vi "Lift state machine.vi"(10 "Grabber Height":dbl, 11 "Joystick Buttons":T2) -> (3 "Motor speed":dbl)   [LabVIEW 2014]
uses:
  Lift state.ctl
  Joystick Buttons typedef.ctl
panel:
  in  "Level setpoints":dbl[](array[numeric])
  in  "Destination":T1
  in  "Direction":enum16{"Not in motion", "Down", "Up"}(ring)
  in  "Lift state":T1
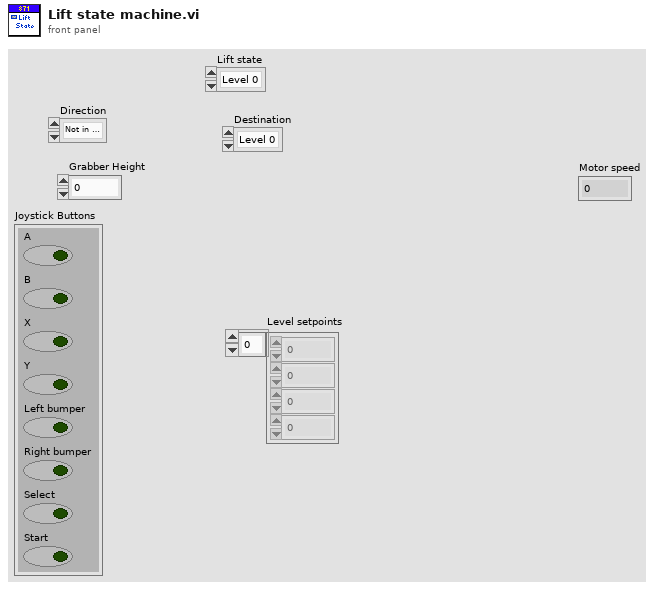
[diagram p1: front panel]
types:
  T1 = typedef "Lift state.ctl" = enum16{"Level 0", "Level 1", "Level 2", "level 3", "Placement State"}
  T2 = typedef "Joystick Buttons typedef.ctl" = cluster{"A":bool, "B":bool, "X":bool, "Y":bool, "Left bumper":bool, "Right bumper":bool, "Select":bool, "Start":bool}
  T3 = typedef "WPI_DigitalInputDevRef.ctl" = cluster{"DevStatus":errorcluster, "DIO Channel":T4, "Controller":T5}
  T4 = typedef "FPGA_DIOChannel.ctl" = enum8{"DIO 0", "DIO 1", "DIO 2", "DIO 3", "DIO 4", "DIO 5", "DIO 6", "DIO 7", "DIO 8", "DIO 9", "DIO MXP 0", "DIO MXP 1", "DIO MXP 2", "DIO MXP 3", "DIO MXP 4", "DIO MXP 5", "DIO MXP 6", "DIO MXP 7", "DIO MXP 8", "DIO MXP 9", "DIO MXP 10", "DIO MXP 11", "DIO MXP 12", "DIO MXP 13", "DIO MXP 14", "DIO MXP 15", "Invalid"}
  T5 = typedef "FPGA_TypedefDigitalModule.ctl" = enum16{"Controller 1"}
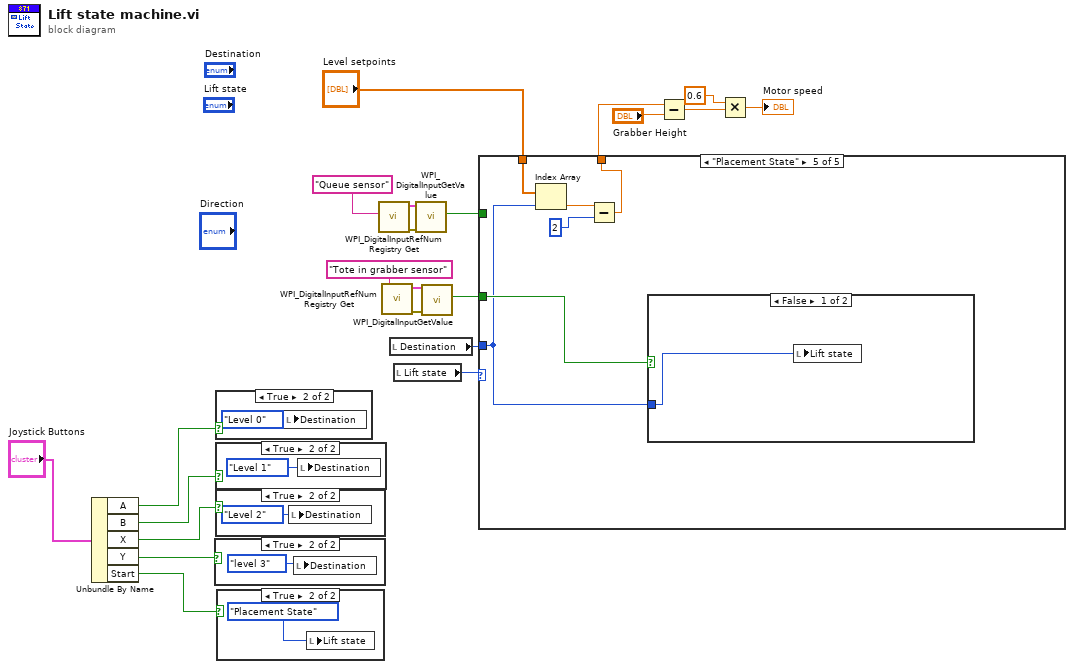
[diagram p0: block diagram]
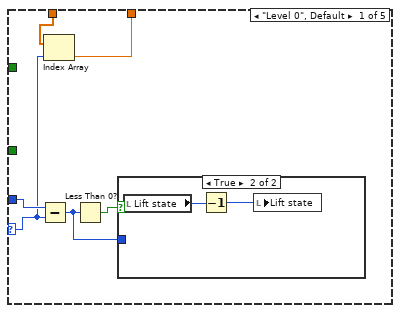
[diagram p7: hidden frame]
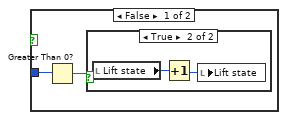
[diagram p8: hidden frame]
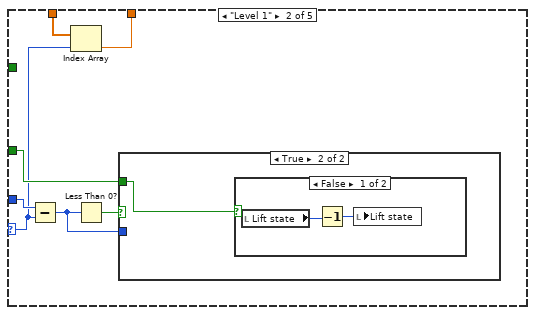
[diagram p10: hidden frame]
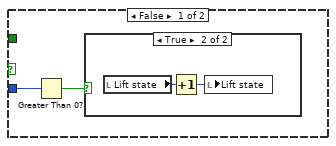
[diagram p11: hidden frame]
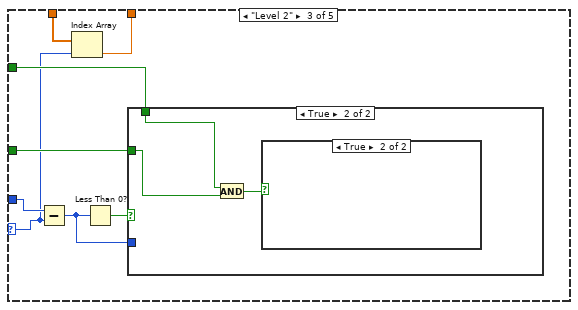
[diagram p14: hidden frame]
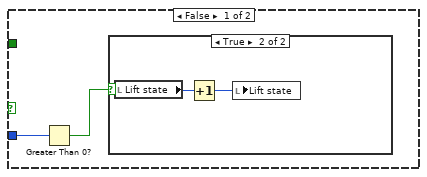
[diagram p15: hidden frame]
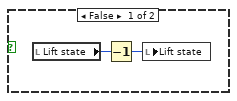
[diagram p17: hidden frame]
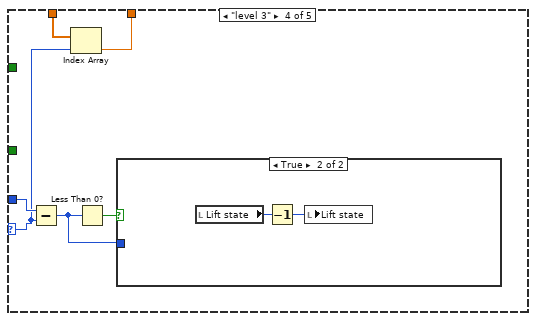
[diagram p18: hidden frame]
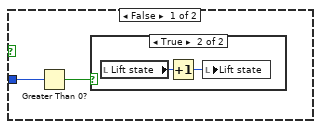
[diagram p19: hidden frame]
diagram:
  n1 = Unbundle By Name("Joystick Buttons") -> ("A"=w10:bool, "B"=w9:bool, "X"=w3:bool, "Y"=w8:bool, "Start"=w2:bool)
  n2 = case shown="True" w8 {
    frame False {
    }
    frame True {
      n3 = local write "Destination"(Lift_state."level 3" ("Lift state")) -> ()
    }
  }
  n4 = case shown="True" w10 {
    frame False {
    }
    frame True {
      n5 = local write "Destination"(Lift_state."Level 0" ("Lift state")) -> ()
    }
  }
  n6 = case shown="True" w9 {
    frame False {
    }
    frame True {
      n7 = local write "Destination"(Lift_state."Level 1" ("Lift state")) -> ()
    }
  }
  n8 = case shown="True" w3 {
    frame False {
    }
    frame True {
      n9 = local write "Destination"(Lift_state."Level 2" ("Lift state")) -> ()
    }
  }
  n10 = case shown="True" w2 {
    frame False {
    }
    frame True {
      n11 = local write "Lift state"(Lift_state."Placement State" ("Lift state")) -> ()
    }
  }
  n12 = call <vilib>:"WPI_DigitalInputRefNum Registry Get.vi"("refnum name"="Queue sensor") -> ("error out"=w7:errorcluster, "DigitalInputDevRef"=w6:T3)  [unwired: 9 in]
  n13 = call <vilib>:"WPI_DigitalInputRefNum Registry Get.vi"("refnum name"="Tote in grabber sensor") -> ("error out"=w15:errorcluster, "DigitalInputDevRef"=w14:T3)  [unwired: 9 in]
  n14 = local read "Destination"() -> (w11:T1)
  n15 = local read "Lift state"() -> (w21:T1)
  n16 = call <vilib>:"WPI_DigitalInputGetValue.vi"("error in (no error)"=w7, "DigitalInputDevRef"=w6) -> ("Value"=w4:bool)  [unwired: 7 in, 2 out]
  n17 = call <vilib>:"WPI_DigitalInputGetValue.vi"("error in (no error)"=w15, "DigitalInputDevRef"=w14) -> ("Value"=w12:bool)  [unwired: 7 in, 2 out]
  n18 = case shown="\"Placement State\"" w21 {
    selector: w21 -> [w28 w40 w54 w71 _]
    tunnel: [w30 w42 w56 w73 w85] -> w19
    tunnel: w12 -> [_ w43 w57 _ w84]
    tunnel: w11 -> [w33 w46 w59 w74 w83]
    tunnel: w4 -> [_ _ w58 _ _]
    tunnel: "Level setpoints" -> [w29 w41 w55 w72 w87]
    frame "Level 0", Default {
      n19 = Subtract(x=w33, y=w28) -> (x-y=w31:u16)
      n20 = Index Array(array=w29, index=w28) -> (element=w30:dbl)
      n21 = Less Than 0?(x=w31) -> (x < 0?=w32:bool)
      n22 = case shown="True" w32 {
        tunnel: w31 -> [w35 _]
        frame False {
          n23 = Greater Than 0?(x=w35) -> (x > 0?=w34:bool)
          n24 = case shown="True" w34 {
            frame False {
            }
            frame True {
              n25 = local read "Lift state"() -> (w37:T1)
              n26 = Increment(x=w37) -> (x+1=w36:T1)
              n27 = local write "Lift state"(w36) -> ()
            }
          }
        }
        frame True {
          n28 = local read "Lift state"() -> (w39:T1)
          n29 = Decrement(x=w39) -> (x-1=w38:T1)
          n30 = local write "Lift state"(w38) -> ()
        }
      }
    }
    frame "Level 1" {
      n31 = Subtract(x=w46, y=w40) -> (x-y=w44:u16)
      n32 = Index Array(array=w41, index=w40) -> (element=w42:dbl)
      n33 = Less Than 0?(x=w44) -> (x < 0?=w45:bool)
      n34 = case shown="True" w45 {
        tunnel: w44 -> [w48 _]
        tunnel: w43 -> [_ w51]
        frame False {
          n35 = Greater Than 0?(x=w48) -> (x > 0?=w47:bool)
          n36 = case shown="True" w47 {
            frame False {
            }
            frame True {
              n37 = local read "Lift state"() -> (w50:T1)
              n38 = Increment(x=w50) -> (x+1=w49:T1)
              n39 = local write "Lift state"(w49) -> ()
            }
          }
        }
        frame True {
          n40 = case shown="False" w51 {
            frame False {
              n41 = local read "Lift state"() -> (w53:T1)
              n42 = Decrement(x=w53) -> (x-1=w52:T1)
              n43 = local write "Lift state"(w52) -> ()
            }
            frame True {
            }
          }
        }
      }
    }
    frame "Level 2" {
      n44 = Subtract(x=w59, y=w54) -> (x-y=w60:u16)
      n45 = Index Array(array=w55, index=w54) -> (element=w56:dbl)
      n46 = Less Than 0?(x=w60) -> (x < 0?=w61:bool)
      n47 = case shown="True" w61 {
        tunnel: w60 -> [w63 _]
        tunnel: w58 -> [_ w66]
        tunnel: w57 -> [_ w67]
        frame False {
          n48 = Greater Than 0?(x=w63) -> (x > 0?=w62:bool)
          n49 = case shown="True" w62 {
            frame False {
            }
            frame True {
              n50 = local read "Lift state"() -> (w65:T1)
              n51 = Increment(x=w65) -> (x+1=w64:T1)
              n52 = local write "Lift state"(w64) -> ()
            }
          }
        }
        frame True {
          n53 = And(x=w66, y=w67) -> (x .and. y?=w68:bool)
          n54 = case shown="True" w68 {
            frame False {
              n55 = local read "Lift state"() -> (w70:T1)
              n56 = Decrement(x=w70) -> (x-1=w69:T1)
              n57 = local write "Lift state"(w69) -> ()
            }
            frame True {
            }
          }
        }
      }
    }
    frame "level 3" {
      n58 = Subtract(x=w74, y=w71) -> (x-y=w75:u16)
      n59 = Index Array(array=w72, index=w71) -> (element=w73:dbl)
      n60 = Less Than 0?(x=w75) -> (x < 0?=w76:bool)
      n61 = case shown="True" w76 {
        tunnel: w75 -> [w78 _]
        frame False {
          n62 = Greater Than 0?(x=w78) -> (x > 0?=w77:bool)
          n63 = case shown="True" w77 {
            frame False {
            }
            frame True {
              n64 = local read "Lift state"() -> (w80:T1)
              n65 = Increment(x=w80) -> (x+1=w79:T1)
              n66 = local write "Lift state"(w79) -> ()
            }
          }
        }
        frame True {
          n67 = local read "Lift state"() -> (w82:T1)
          n68 = Decrement(x=w82) -> (x-1=w81:T1)
          n69 = local write "Lift state"(w81) -> ()
        }
      }
    }
    frame "Placement State" {
      n70 = Index Array(array=w87, index=w83) -> (element=w88:dbl)
      n71 = Subtract(x=w88, y=2) -> (x-y=w85:dbl)
      n72 = case shown="False" w84 {
        tunnel: w83 -> [w89 _]
        frame False {
          n73 = local write "Lift state"(w89) -> ()
        }
        frame True {
        }
      }
    }
  }
  n74 = Subtract(x=w19, y="Grabber Height") -> (x-y=w17:dbl)
  n75 = Multiply(x=0.6, y=w17) -> (x*y=→"Motor speed":dbl)
